vi "Bus Load Calculation.vi"(8 "error in":errorcluster, 9 "Current Iteration":i32, 10 "millisecond timer value in":u32, 11 "NewData":bool) -> (0 "error out":errorcluster, 1 "BusLoad":dbl, 2 "millisecond timer value out":u32, 3 "Peak Bus Load":dbl)   [LabVIEW 2014, in "CAN Bus Monitor Engine.lvlib"]
uses:
  CAN Bus Monitor Engine.lvlib
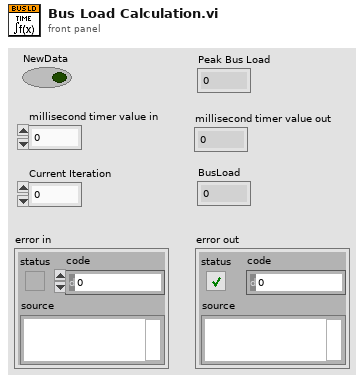
[diagram p1: front panel]
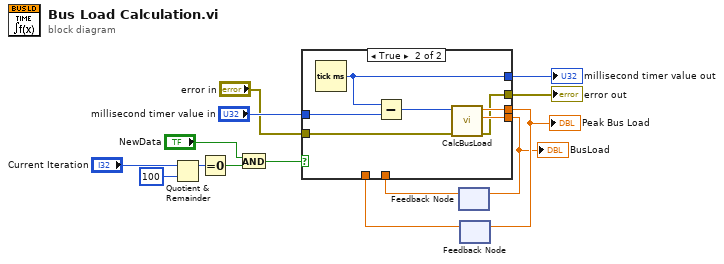
[diagram p0: block diagram]
diagram:
  n1 = Quotient & Remainder(x="Current Iteration", y=100) -> (x-y*floor(x/y)=w5:i32)  [unwired: 1 out]
  n2 = Equal To 0?(x=w5) -> (x = 0?=w6:bool)
  n3 = And(x="NewData", y=w6) -> (x .and. y?=w7:bool)
  n4 = feedback #1() -> (w9:dbl)  [unwired: 1 in]
  n5 = feedback #2() -> (w14:dbl)  [unwired: 1 in]
  n6 = case shown="True" w7 {
    tunnel: [w18 w25] -> w8
    tunnel: w9 -> [w18 _]
    tunnel: "millisecond timer value in" -> [w17 w24]
    tunnel: [w17 w23] -> w11
    tunnel: [w16 w21] -> w13
    tunnel: w14 -> [w16 _]
    tunnel: [w15 w20] -> w2
    tunnel: "error in" -> [w15 w19]
    frame False {
    }
    frame True {
      n7 = Tick Count (ms)() -> (millisecond timer value=w23:u32)
      n8 = Subtract(x=w23, y=w24) -> (x-y=w22:u32)
      n9 = call "CalcBusLoad.vi"("error in"=w19, "UpdateDelay [ms]"=w22) -> ("error out"=w20:errorcluster, "BusLoad"=w25:dbl, "Peak Bus Load"=w21:dbl)  [unwired: 7 in]
    }
  }
  "Peak Bus Load" <- w13
  "millisecond timer value out" <- w11
  "BusLoad" <- w8
  "error out" <- w2
  n10 = feedback-in #1(w8) -> ()
  n11 = feedback-in #2(w13) -> ()
